vi "Roller Logic.vi"(8 "error in (no error)":errorcluster, 10 "Roller Input Data":T1) -> (0 "error out":errorcluster, 2 "Right motor":dbl, 3 "Left Motor":dbl)   [LabVIEW 2014]
uses:
  Roller Input Data.ctl
  Utilities/Rising Edge Detector.vi
panel:
  in  "Feeder Roller Speed":dbl=-0.5
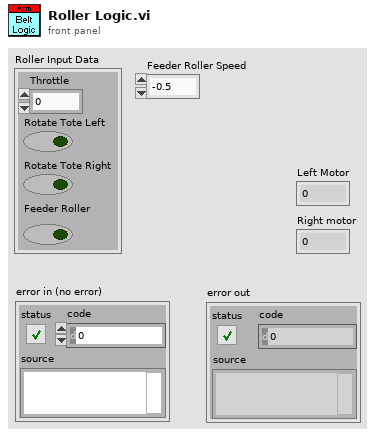
[diagram p1: front panel]
types:
  T1 = typedef "Roller Input Data.ctl" = cluster{"Throttle":dbl, "Rotate Tote Left":bool, "Rotate Tote Right":bool, "Feeder Roller":bool}
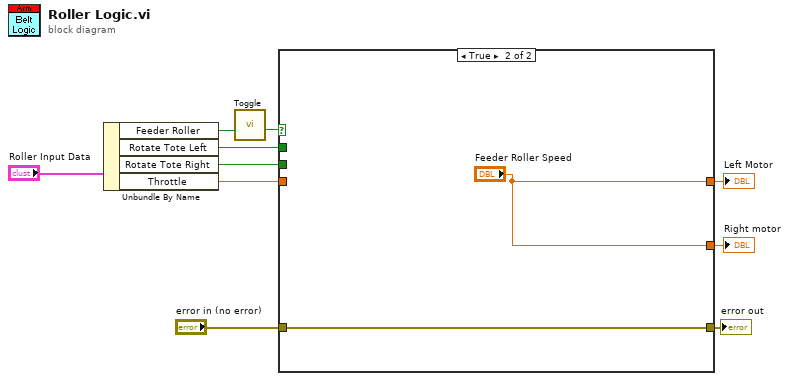
[diagram p0: block diagram]
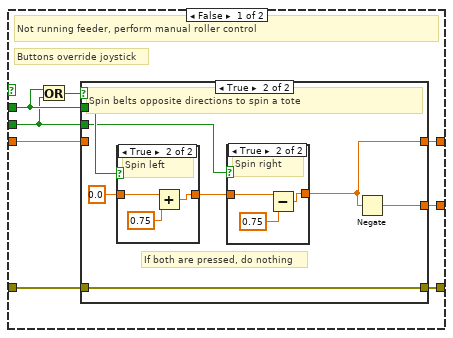
[diagram p2: hidden frame]
diagram:
  n1 = Unbundle By Name("Roller Input Data") -> ("Feeder Roller"=w2:bool, "Rotate Tote Left"=w7:bool, "Rotate Tote Right"=w6:bool, "Throttle"=w9:dbl)
  n2 = call "Toggle.vi"("Input"=w2) -> ("Toggled output"=w1:bool)  [unwired: 10 in]
  n3 = case shown="True" w1 {
    tunnel: w9 -> [w18 _]
    tunnel: [w17 "Feeder Roller Speed"] -> w8
    tunnel: w7 -> [w15 _]
    tunnel: w6 -> [w14 _]
    tunnel: [w13 "Feeder Roller Speed"] -> w5
    tunnel: "error in (no error)" -> [w12 w36]
    tunnel: [w11 w36] -> w3
    frame False {
      # "Buttons override joystick"
      # "Not running feeder, perform manual roller control"
      n4 = Or(x=w15, y=w14) -> (x .or. y?=w16:bool)
      n5 = case shown="True" w16 {
        tunnel: w18 -> [w20 _]
        tunnel: [w20 w27] -> w17
        tunnel: w15 -> [_ w23]
        tunnel: w14 -> [_ w22]
        tunnel: [w20 w24] -> w13
        tunnel: w12 -> [w19 w21]
        tunnel: [w19 w21] -> w11
        frame False {
          # "Pass through joystick value"
        }
        frame True {
          # "If both are pressed, do nothing"
          # "Spin belts opposite directions to spin a tote"
          n6 = case shown="True" w23 {
            tunnel: 0.0 -> [w32 w34]
            tunnel: [w32 w33] -> w25
            frame False {
            }
            frame True {
              # "Spin left"
              n7 = Add(x=w34, y=0.75) -> (x+y=w33:dbl)
            }
          }
          n8 = case shown="True" w22 {
            tunnel: w25 -> [w28 w31]
            tunnel: [w28 w29] -> w24
            frame False {
            }
            frame True {
              # "Spin right"
              n9 = Subtract(x=w31, y=0.75) -> (x-y=w29:dbl)
            }
          }
          n10 = Negate(x=w24) -> (-x=w27:dbl)
        }
      }
    }
    frame True {
    }
  }
  "Left Motor" <- w5
  "Right motor" <- w8
  "error out" <- w3
